vi "Send cmd S4ICS.vi"(8 "error in (no error)":errorcluster, 9 "port":u16, 10 "address":string, 11 "data in":string) -> (0 "error out":errorcluster, 3 "data out":string)   [LabVIEW 2018]
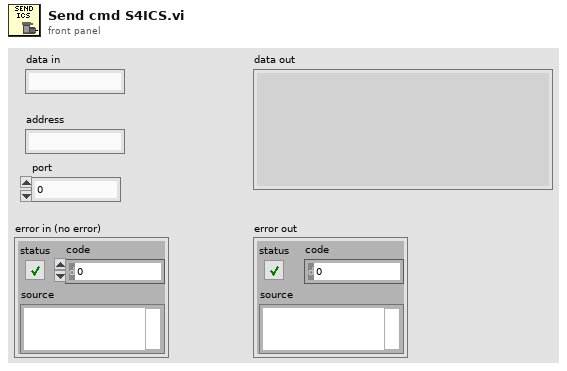
[diagram p1: front panel]
types:
  T1 = enum16{"Standard", "Buffered", "CRLF", "Immediate"}
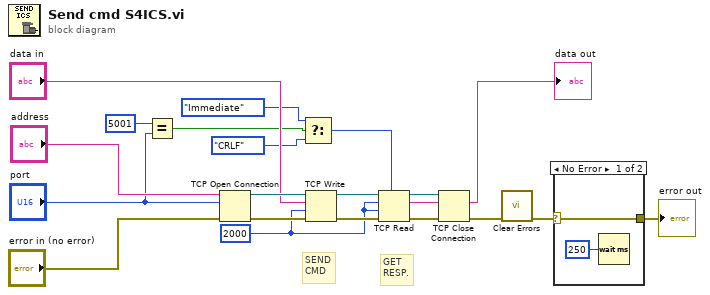
[diagram p0: block diagram]
diagram:
  w15 = 2000 ("bytes to read")
  # "GET\nRESP."
  # "SEND\nCMD"
  n1 = Equal?(x=u16 5001, y="port") -> (x = y?=w7:bool)
  n2 = TCP Open Connection(address="address", remote port or service name="port", error in (no error)="error in (no error)") -> (connection ID=w20:refnum<k5>, error out=w19:errorcluster)  [unwired: 2 out]
  n3 = Select(t=T1."Immediate" ("mode (standard)"), s=w7, f=T1."CRLF" ("mode (standard)")) -> (s? t:f=w6:T1)
  n4 = TCP Write(connection ID=w20, data in="data in", error in (no error)=w19, 9:w15) -> (connection ID out=w17:refnum<k5>, error out=w16:errorcluster)  [unwired: 1 out]
  n5 = TCP Read(connection ID=w17, bytes to read=w15, error in (no error)=w16, 7:w6, 9:w15) -> (connection ID out=w11:refnum<k5>, data out=→"data out":string, error out=w10:errorcluster)
  n6 = TCP Close Connection(connection ID=w11, error in (no error)=w10) -> (error out=w3:errorcluster)  [unwired: 1 in, 1 out]
  n7 = call <vilib>:"Clear Errors.vi"("error in (no error)"=w3) -> ("error out"=w2:errorcluster)  [unwired: 5 in, 1 out]
  n8 = case shown="No Error" w2 {
    selector: w2 -> [w22 w23]
    tunnel: [w22 w23] -> w1
    frame No Error {
      n9 = Wait (ms)(milliseconds to wait=u32 250) -> ()  [unwired: 1 out]
    }
    frame Error {
    }
  }
  "error out" <- w1
